vi "LinearScaling.vi"(1 "b":dbl, 2 "a":dbl, 3 "X":dbl) -> (0 "y":dbl)   [LabVIEW 2021]
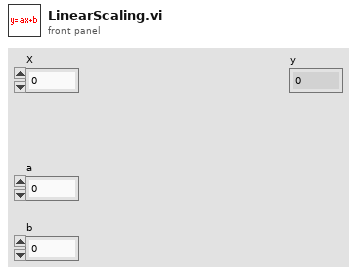
[diagram p1: front panel]
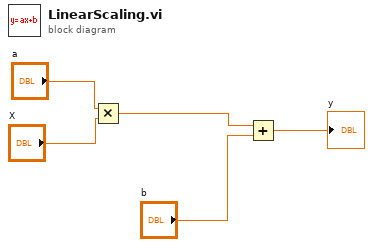
[diagram p0: block diagram]
diagram:
  n1 = Multiply(x="a", y="X") -> (x*y=w2:dbl)
  n2 = Add(x=w2, y="b") -> (x+y=→"y":dbl)
